vi "VMS_Test.vi"() -> ()   [LabVIEW 2016]
uses:
  <vilib>/rvi/eio/common/nirviEmuTemplateMethod_errors.vi
  <vilib>/rvi/Emulation/niFpgaGetClockAttributes.vi
  <vilib>/rvi/Emulation/niFpgaSctlEmulationGetInTimedLoop.vi
  <vilib>/rvi/Emulation/niFpgaEmulationReportErrorSimple.vi
  <vilib>/rvi/Emulation/niFpgaCriticalErrorInLSC.vi
  <vilib>/eio/EIONode/EIONode.xnode
panel:
  out "single precision float 3":sgl format="%.6f"
  out "single precision float 2":sgl format="%.6f"
  out "single precision float":sgl format="%.6f"
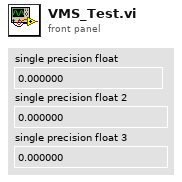
[diagram p1: front panel]
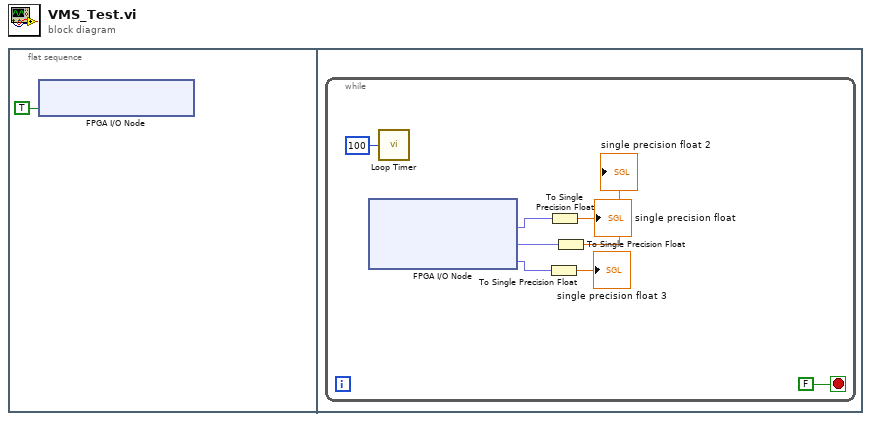
[diagram p0: block diagram]
diagram:
  n1 = flat-sequence {
    frame #0 {
      n2 = xnode "FPGA I/O Node"("Accelerometer1/Start"=TRUE) -> ()  [unwired: 1 in, 1 out]
    }
    frame #1 {
      n3 = while {
        stop <- FALSE stop-if-true
        n4 = xnode "FPGA I/O Node"() -> ("Accelerometer1/AI0"=w5:fxp<+/-,24,7>, "Accelerometer1/AI1"=w6:fxp<+/-,24,7>, "Accelerometer1/AI2"=w7:fxp<+/-,24,7>)  [unwired: 3 in, 3 out]
        n5 = call "Loop Timer"("Count(mSec)"=u32 100) -> ()  [unwired: 1 out]
        n6 = To Single Precision Float(number=w7) -> (single precision float=→"single precision float 3":sgl)
        n7 = To Single Precision Float(number=w5) -> (single precision float=→"single precision float":sgl)
        n8 = To Single Precision Float(number=w6) -> (single precision float=→"single precision float 2":sgl)
      }
    }
  }
